vi "x squared normal.vi"(11 "x":dbl) -> (3 "nearest integer value":dbl)   [LabVIEW 2013]
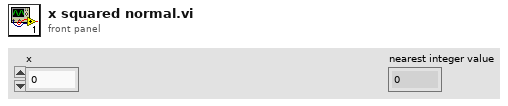
[diagram p1: front panel]
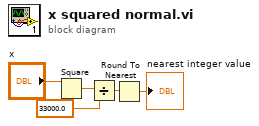
[diagram p0: block diagram]
diagram:
  n1 = Square(x="x") -> (x^2=w3:dbl)
  n2 = Divide(x=w3, y=33000.0) -> (x/y=w4:dbl)
  n3 = Round To Nearest(number=w4) -> (nearest integer value=→"nearest integer value":dbl)
